vi "Run Measurement.vi"(6 "Show FP?":bool=TRUE, 8 "error in (no error)":errorcluster, 9 "Device Names":string[](array[string]), 10 "Measurement Name":string, 11 "Self Enqueuer In":refnum<class "Message Enqueuer.lvclass">) -> (0 "error out":errorcluster, 2 "Measurement Results":refnum<class "Results.lvclass">, 3 "Self Enqueuer Out":refnum<class "Message Enqueuer.lvclass">)   [LabVIEW 2016, in "Controller API.lvlib" / "Controller API.lvclass"]
uses:
  <userlib>/Measurement Utility API/Controller API.lvclass
  <vilib>/ActorFramework/Message Enqueuer/Message Enqueuer.lvclass
  <userlib>/Common Components/Results/Results.lvclass
  <userlib>/Measurement Utility API/Messages/Launch Measurement Msg/Launch Measurement and Wait for Result.lvclass
  C:/Program Files (x86)/National Instruments/LabVIEW 2016/user.lib/Common Components/Controller/Messages/Launch Measurements Message/Launch Measurements Message.lvclass
  C:/Program Files (x86)/National Instruments/LabVIEW 2016/vi.lib/ActorFramework/Message/Message.lvclass
  <userlib>/Measurement Utility API/Error Result/Error Report.lvclass
  <userlib>/Common Components/Controller/Messages/Launch Measurements Message/Launch Measurements Message.lvclass/Launch Measurements Message.ctl
  <userlib>/Measurement Utility API/Messages/Launch Measurement Msg/Launch Measurement and Wait for Result.lvclass/Launch Measurement and Wait for Result.ctl
  <vilib>/ActorFramework/Message Enqueuer/Message Enqueuer.lvclass/Message Enqueuer.ctl
  <userlib>/Measurement Utility API/Error Result/Error Report.lvclass/Error Report.ctl
  <vilib>/ActorFramework/Message Priority Queue/Priority Enqueue.vi
  <userlib>/Common Components/Controller/Messages/Launch Measurements Message/Launch Measurements Message.lvclass
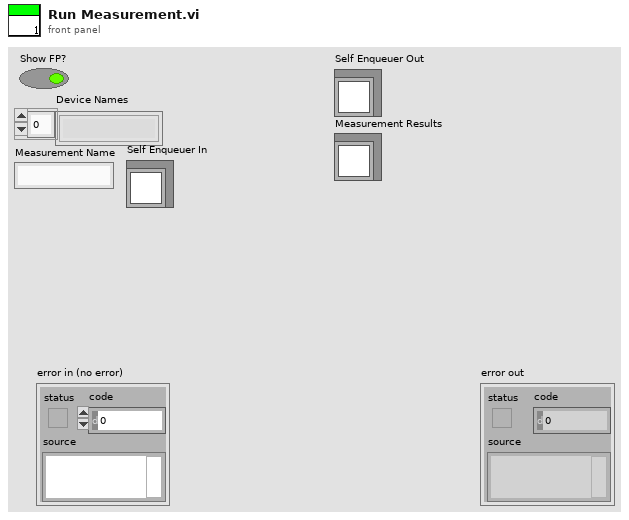
[diagram p1: front panel]
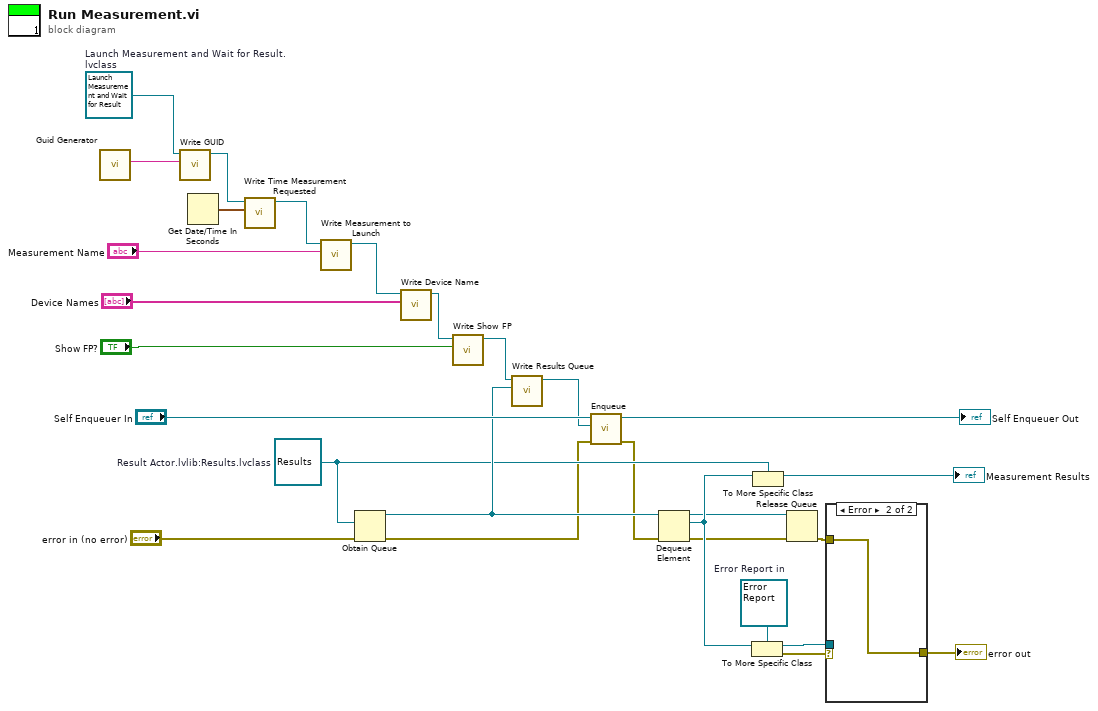
[diagram p0: block diagram]
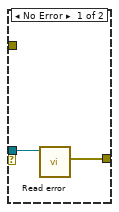
[diagram p2: hidden frame]
diagram:
  w9 = refnum<class "Error Report.lvclass"> refnum  # Error Report in
  w1 = refnum<class "Launch Measurement and Wait for Result.lvclass"> refnum  # Launch Measurement and Wait for Result.lvclass
  w5 = refnum<class "Results.lvclass"> refnum  # Result Actor.lvlib:Results.lvclass
  n1 = call <vilib>:"Guid Generator.vi"() -> ("GUID"=w14:string)  [unwired: 10 in, 1 out]
  n2 = call <userlib>:"Write GUID.vi"("GUID"=w14, "Launch Measurements Message in"=w1) -> ("Launch Measurements Message out"=w15:refnum<class "Launch Measurement and Wait for Result.lvclass">)  [unwired: 8 in, 1 out]
  n3 = Get Date/Time In Seconds() -> (seconds since 1Jan1904=w16:timestamp)
  n4 = call <userlib>:"Write Time Measurement Requested.vi"("Time Measurement Requested"=w16, "Launch Measurements Message in"=w15) -> ("Launch Measurements Message out"=w17:refnum<class "Launch Measurement and Wait for Result.lvclass">)  [unwired: 8 in, 1 out]
  n5 = call <userlib>:"Write Measurement to Launch.vi"("Measurement Name"="Measurement Name", "Launch Measurements Message in"=w17) -> ("Launch Measurements Message out"=w26:refnum<class "Launch Measurement and Wait for Result.lvclass">)  [unwired: 8 in, 1 out]
  n6 = Obtain Queue(element data type=w5, error in (no error)="error in (no error)") -> (queue out=w23:refnum<queue>, error out=w4:errorcluster)  [unwired: 3 in, 1 out]
  n7 = call <userlib>:"Write Device Name.vi"("Device Names"="Device Names", "Launch Measurements Message in"=w26) -> ("Launch Measurements Message out"=w25:refnum<class "Launch Measurement and Wait for Result.lvclass">)  [unwired: 8 in, 1 out]
  n8 = call <userlib>:"Write Show FP.vi"("Show FP?"="Show FP?", "Launch Measurements Message in"=w25) -> ("Launch Measurements Message out"=w24:refnum<class "Launch Measurement and Wait for Result.lvclass">)  [unwired: 8 in, 1 out]
  n9 = call <userlib>:"Write Results Queue.vi"("Results Queue"=w23, "Launch Measurement and Wait for Result in"=w24) -> ("Launch Measurement and Wait for Result out"=w19:refnum<class "Launch Measurement and Wait for Result.lvclass">)  [unwired: 8 in, 1 out]
  n10 = call <vilib>:"Enqueue.vi"("error in (no error)"=w4, "Message"=w19, "Message Enqueuer in"="Self Enqueuer In") -> ("error out"=w3:errorcluster, "Message Enqueuer out"=→"Self Enqueuer Out":refnum<class "Message Enqueuer.lvclass">)  [unwired: 7 in]
  n11 = Dequeue Element(queue=w23, error in (no error)=w3) -> (queue out=w7:refnum<queue>, element=w12:refnum<class "Results.lvclass">, error out=w6:errorcluster)  [unwired: 1 in, 1 out]
  n12 = To More Specific Class(target class=w9, reference=w12) -> (specific class reference=w8:refnum<class "Error Report.lvclass">, error out=w11:errorcluster)  [unwired: 1 in]
  n13 = To More Specific Class(target class=w5, reference=w12) -> (specific class reference=→"Measurement Results":refnum<class "Results.lvclass">)  [unwired: 1 in, 1 out]
  n14 = Release Queue(queue=w7, error in (no error)=w6) -> (error out=w2:errorcluster)  [unwired: 1 in, 2 out]
  n15 = case shown="Error" w11 {
    tunnel: w8 -> [w30 _]
    tunnel: [w29 w31] -> w10
    tunnel: w2 -> [_ w31]
    frame No Error {
      n16 = call <userlib>:"Read error.vi"("Error Report in"=w30) -> ("error"=w29:errorcluster)  [unwired: 8 in, 2 out]
    }
    frame Error {
    }
  }
  "error out" <- w10
